vi "Read Trace Data Statistic.vi"(8 "error in (no error)":errorcluster, 9 "Statistical Operation (4: Mean)":i32(ring)=4 items=["Minimum", "Maximum", "Standard Deviation", "Peak To Peak", "Mean"], 10 "Channel (1: Channel 1)":i32(ring)=1 items=["Channel 1"=1, "Channel 2"=2], 11 "VISA resource name":refnum<visa-resource-name>) -> (0 "error out":errorcluster, 2 "Trace Data Statistical Result":dbl, 3 "VISA resource name out":refnum<visa-resource-name>)   [LabVIEW 2012, in "Keysight B2980 Series.lvlib"]
doc: "Returns the result of the statistical operation for the data stored in the trace buffer."
uses:
  Keysight B2980 Series.lvlib
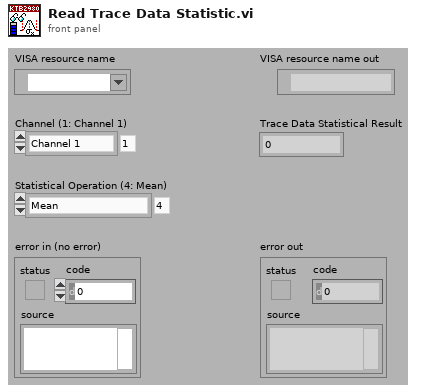
[diagram p1: front panel]
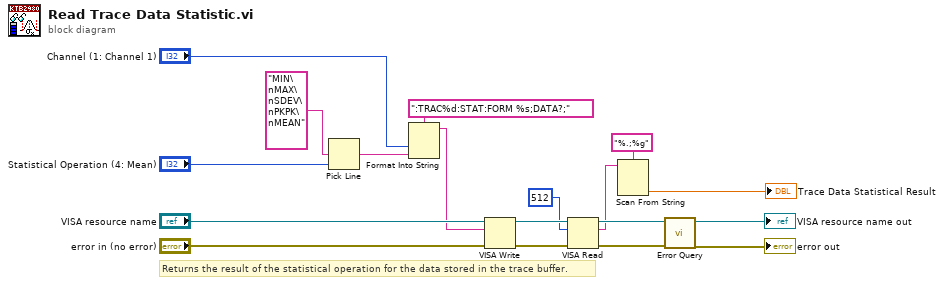
[diagram p0: block diagram]
diagram:
  # "Returns the result of the statistical operation for the data stored in the trace buffer."
  n1 = Pick Line(multi-line string="MIN\nMAX\nSDEV\nPKPK\nMEAN", line index="Statistical Operation (4: Mean)") -> (output string=w14:string)  [unwired: 1 out]
  n2 = Format Into String(format string=":TRAC%d:STAT:FORM %s;DATA?;", "Channel (1: Channel 1)", w14) -> (resulting string=w1:string)  [unwired: 2 in, 1 out]
  n3 = VISA Write(VISA resource name="VISA resource name", write buffer=w1, error in (no error)="error in (no error)") -> (VISA resource name out=w9:refnum<visa-resource-name>, error out=w8:errorcluster)  [unwired: 1 out]
  n4 = VISA Read(VISA resource name=w9, byte count=u32 512, error in (no error)=w8) -> (VISA resource name out=w7:refnum<visa-resource-name>, read buffer=w4:string, error out=w6:errorcluster)  [unwired: 1 out]
  n5 = Scan From String(format string="%.;%g", input string=w4) -> (output 1=→"Trace Data Statistical Result":dbl)  [unwired: 2 in, 4 out]
  n6 = call "Error Query.vi"("error in (no error)"=w6, "VISA resource name"=w7) -> ("error out"=→"error out":errorcluster, "VISA resource name out"=→"VISA resource name out":refnum<visa-resource-name>)  [unwired: 8 out]
